vi "Show Context Buttons.vi"(8 "error in (no error)":errorcluster, 9 "Coords":T1, 11 "Refs":T2) -> (0 "error out":errorcluster)   [LabVIEW 2020, in "MacroAssert.lvlib"]
doc: "Shows the context buttons for editing steps after the steps list has been double clicked."
uses:
  MacroAssert.lvlib
  CTLs/Refs.ctl
  <vilib>/Utility/miscctls.llb/LVPoint32TypeDef.ctl
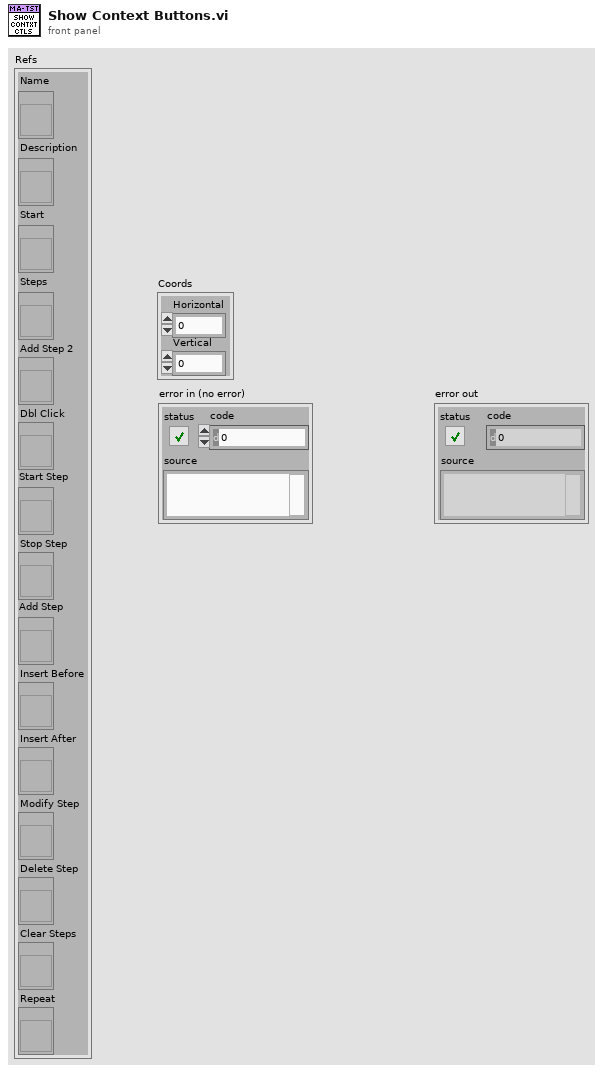
[diagram p1: front panel]
types:
  T1 = typedef "LVPoint32TypeDef.ctl" = cluster{"Horizontal":i32, "Vertical":i32}
  T2 = typedef "MacroAssert.lvlib/Refs.ctl" = cluster{"Name":refnum<vi>, "Description":refnum<vi>, "Start":refnum<vi>, "Steps":refnum<vi>, "Add Step 2":refnum<vi>, "Dbl Click":refnum<vi>, "Start Step":refnum<vi>, "Stop Step":refnum<vi>, "Add Step":refnum<vi>, "Insert Before":refnum<vi>, "Insert After":refnum<vi>, "Modify Step":refnum<vi>, "Delete Step":refnum<vi>, "Clear Steps":refnum<vi>, "Repeat":refnum<vi>}
  T3 = typedef "LVRectTypeDef.ctl" = cluster{"Left":i16, "Top":i16, "Right":i16, "Bottom":i16}
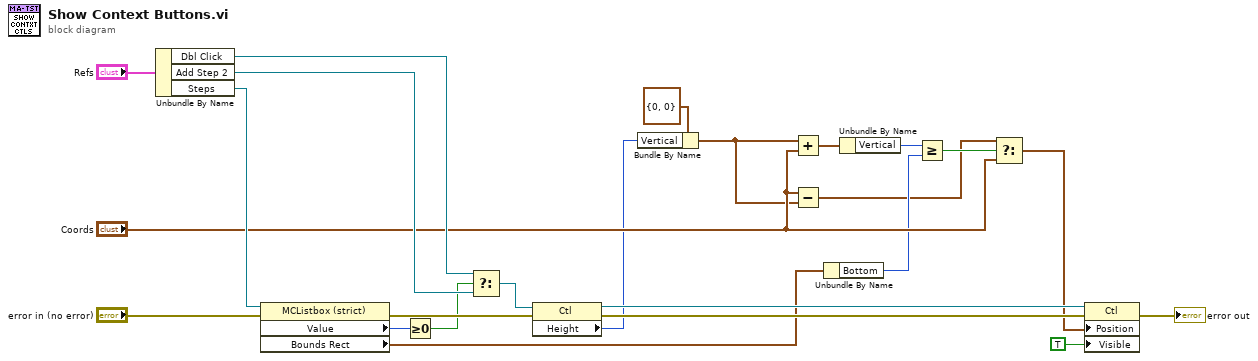
[diagram p0: block diagram]
diagram:
  n1 = Unbundle By Name("Refs") -> ("Dbl Click"=w18:refnum<vi>, "Add Step 2"=w19:refnum<vi>, "Steps"=w20:refnum<vi>)
  n2 = property on="Property Node" class="MCListbox (strict)"(reference=w20, error in="error in (no error)") -> (error out=w23:errorcluster, "Value"=w1:i32, "Bounds Rect"=w2:T3)  [unwired: 1 out]
  n3 = Greater Or Equal To 0?(x=w1) -> (x >= 0?=w12:bool)
  n4 = Select(t=w18, s=w12, f=w19) -> (s? t:f=w17:refnum<vi>)
  n5 = property on="Property Node" class="Ctl"(reference=w17, error in=w23) -> (reference out=w16:refnum<vi>, error out=w21:errorcluster, "Height"=w4:u32)
  n6 = Bundle By Name(cluster=T1 {"Horizontal"=0, "Vertical"=0} ("Coords"), "Vertical"=w4) -> (w3:T1)
  n7 = Add(x=w3, y="Coords") -> (x+y=w10:T1)
  n8 = Subtract(x="Coords", y=w3) -> (x-y=w7:T1)
  n9 = Unbundle By Name(w2) -> ("Bottom"=w13:i16)
  n10 = Unbundle By Name(w10) -> ("Vertical"=w9:i32)
  n11 = Greater Or Equal?(x=w9, y=w13) -> (x >= y?=w8:bool)
  n12 = Select(t=w7, s=w8, f="Coords") -> (s? t:f=w6:T1)
  n13 = property on="Property Node" class="Ctl"(reference=w16, error in=w21, "Position"=w6, "Visible"=TRUE) -> (error out=→"error out":errorcluster)  [unwired: 1 out]
